vi "Read Read Only.vi"(8 "error in (no error)":errorcluster, 11 "Const_DBL in":refnum<class "Const_DBL_1D.lvclass">) -> (0 "error out":errorcluster, 2 "Read Only":bool, 3 "Const_DBL out":refnum<class "Const_DBL_1D.lvclass">)   [LabVIEW 2021, in "Const_DBL_1D.lvclass"]
uses:
  Const_DBL_1D.lvclass
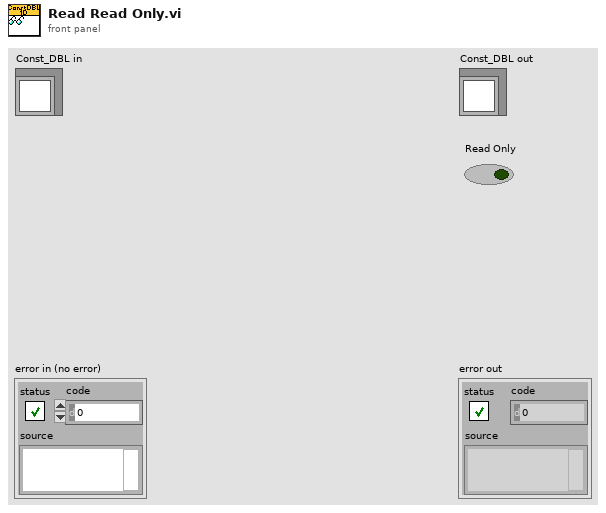
[diagram p1: front panel]
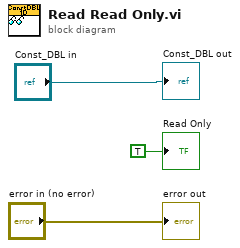
[diagram p0: block diagram]
diagram:
  "error out" <- "error in (no error)"
  "Const_DBL out" <- "Const_DBL in"
  "Read Only" <- TRUE ("Read Only")
